vi "Stand Alone Test - Timer Module - Unpause Timer1.vi"() -> ()   [LabVIEW 2018]
panel:
  out "Final Timer":timestamp format="%^<%H:%M:%S%3u>T"
  out "Pass?":bool
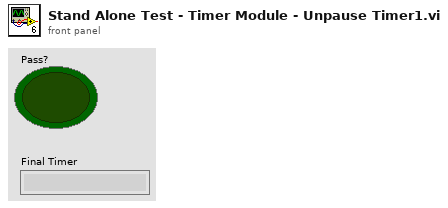
[diagram p1: front panel]
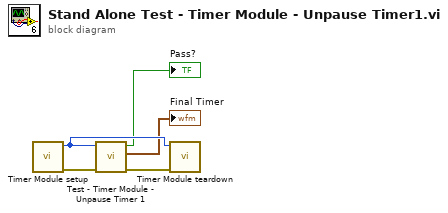
[diagram p0: block diagram]
diagram:
  n1 = call "Timer Module setup.vi"() -> ("error out"=w5:errorcluster, "Module ID"=w3:i32)  [unwired: 10 in]
  n2 = call "Test - Timer Module - Unpause Timer 1.vi"("error in (no error)"=w5, "Module ID"=w3) -> ("error out"=w4:errorcluster, "Final Timer"=→"Final Timer":timestamp, "Pass"=→"Pass?":bool)  [unwired: 7 in]
  n3 = call "Timer Module teardown.vi"("error in (no error)"=w4, "Module ID"=w3) -> ()  [unwired: 9 in, 1 out]
